vi "load_array_of_boxes_xml.vi"(8 "error in":errorcluster, 11 "node in":refnum<k20>) -> (0 "error out":errorcluster, 2 "ArrayOfDDSBoxes":T1[](array[typedef]) {"Array of DDS Channels (4)"."Array of DDS Profiles (8)"."Time Step (us)" min=0.0 max=262.14 step=0.004 format="%8.3g"; "Array of DDS Channels (4)"."Channel Parameters"."Ref Clock Rate [MHz]" min=0.0}, 3 "node":refnum<k20>)   [LabVIEW 2014, in "DDS.lvclass"]
doc: "Loads array of DDS boxes from XML. Expected format:\n\n<box>\n<Enable>%b</Enable>\n<DDSBoxDeviceReference.Resource>%s</DDSBoxDeviceReference.Resource>\n<DDSBoxDeviceReference.DIOPort>%u</DDSBoxDeviceReference.DIOPort>\n<DDSBoxDeviceReference.SerialClockRate units=\"kHz\">%u</DDSBoxDeviceReference.SerialClockRate>\n<ArrayOfDDSChannels>\n\n<channel>\n<Power>%b</Power>\n<ChannelParameters.RefClockRate units=\"kHz\">%f</ChannelParameters.RefClockRate>\n<ChannelParameters.FullScaleOutputPower units=\"dBm\">%f</ChannelParameters.FullScaleOutputPower>\n<RAMEnable>%b</RAMEnable>\n<RAMDestType>%u</RAMDestType>\n<RAMDefault.Frequency units=\"MHz\">%s</RAMDefault.Frequency>\n<RAMDefault.Amplitude units=\"dBm\">%s</RAMDefault.Amplitude>\n<RAMDefault.Phase units=\"rad\">%s</RAMDefault.Phase>\n<ArrayOfDDSProfiles>\n\n<profile>\n<SingleTone.Frequency units=\"MHz\">%s</SingleTone.Frequency>\n<SingleTone.Amplitude units=\"dBm\">%s</SingleTone.Amplitude>\n<SingleTone.Phase units=\"rad\">%s</SingleTone.Phase>\n<RAMMode>%u</RAMMode>\n<ZeroCrossing>%b</ZeroCrossing>\n<NoDwellHigh>%b</NoDwellHigh>\n<FunctionOrStatic>%b</FunctionOrStatic>\n<RAMFunctionSettings>%s</RAMFunctionSettings>\n<RAMStaticArray>%s</RAMStaticArray>\n</profile>\n\n</ArrayOfDDSProfiles>\n</channel>\n\n</ArrayOfDDSChannels>\n</box>\n\nMTL 2012 Dec 31"
uses:
  DDS.lvclass
  DDS Library/Controls/DDS RAM Mode.ctl
  DDS Library/DDS.lvlib
  <vilib>/ni845x/ni845x.llb/ni845xControl.ctl
  DDS Library/Controls/DDS Box Device Reference.ctl
  DDS Library/Controls/DDS Box Cluster.ctl
  <resource>/objmgr/DOMUserDefRef.rc
  <vilib>/xml/NI_XML.lvlib
  <vilib>/xml/Close Reference(Node).vi
  DDS Library/Controls/DDS Profile.ctl
  DDS Library/Controls/DDS Channel.ctl
  DDS Library/Controls/DDS Profile Array.ctl
  DDS Library/Controls/DDS Channel Array.ctl
  DDS Library/Controls/DDS RAM Timestep.ctl
  DDS Library/Controls/DDS RAM Destination.ctl
  DDS Library/Controls/DDS Channel Parameters.ctl
panel:
  # "f/f/A"
  # "Mag"
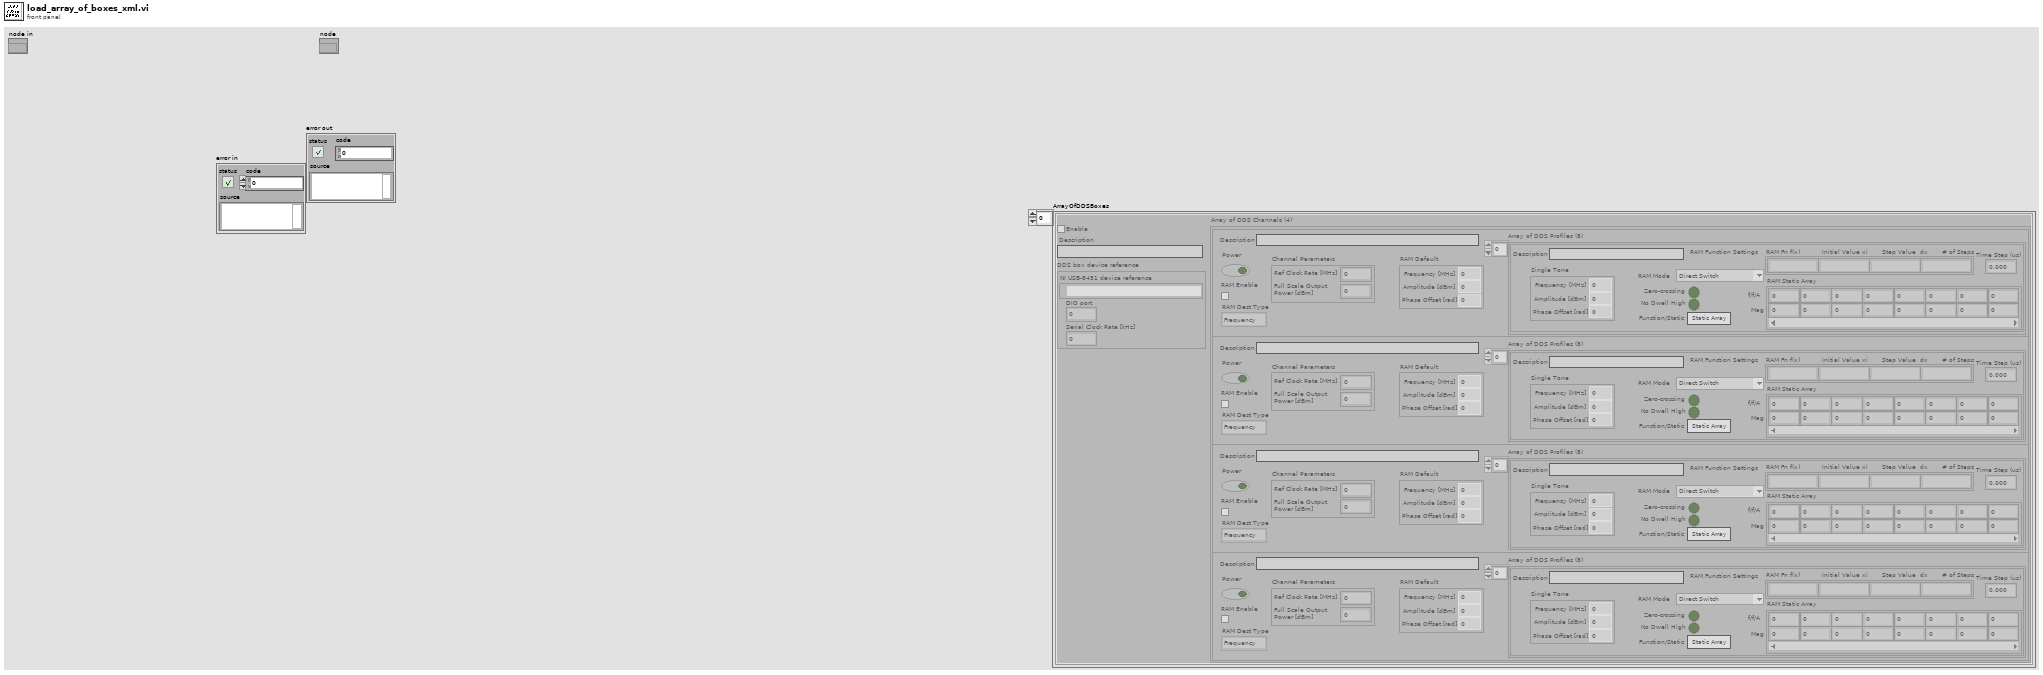
[diagram p1: front panel]
types:
  T1 = typedef "DDS.lvlib/DDS Box Cluster.ctl" = cluster{"DDS box device reference":T2, "Array of DDS Channels (4)":T4, "Enable":bool, "Description":string}
  T2 = typedef "DDS.lvlib/DDS Box Device Reference.ctl" = cluster{"NI USB-8451 device reference":T3, "DIO port":u8, "Serial Clock Rate [kHz]":u16}
  T3 = typedef "ni845xControl.ctl" = refnum<k21>
  T4 = typedef "DDS.lvlib/DDS Channel Array.ctl" = T5[]
  T5 = typedef "DDS.lvlib/DDS Channel.ctl" = cluster{"Power":bool, "Channel Parameters":T6, "RAM Enable":bool, "RAM Dest Type":T7, "RAM Default":cluster{"Frequency [MHz]":dbl, "Amplitude [dBm]":dbl, "Phase Offset [rad]":dbl}, "Array of DDS Profiles (8)":T8, "Description":string}
  T6 = typedef "DDS.lvlib/DDS Channel Parameters.ctl" = cluster{"Ref Clock Rate [MHz]":dbl, "Full Scale Output\nPower [dBm]":dbl}
  T7 = typedef "DDS.lvlib/DDS RAM Destination.ctl" = enum16{"Frequency", "Phase", "Amplitude", "Polar"}
  T8 = typedef "DDS.lvlib/DDS Profile Array.ctl" = T9[]
  T9 = typedef "DDS.lvlib/DDS Profile.ctl" = cluster{"Single Tone":cluster{"Frequency [MHz]":dbl, "Amplitude [dBm]":dbl, "Phase Offset [rad]":dbl}, "RAM Mode ":T10, "Zero-crossing":bool, "No Dwell High":bool, "Function/Static":bool, "RAM Function Settings":string[], "RAM Static Array":dbl[][], "Description":string, "Time Step (us)":T11}
  T10 = typedef "DDS.lvlib/DDS RAM mode.ctl" = enum16{"Direct Switch", "Ramp Up", "Bidirectional Ramp", "Continuous Bidirectional Ramp", "Continuous Recirculate", "Direct Switch 2", "Direct Switch 3", "Direct Switch 4"}
  T11 = typedef "DDS.lvlib/DDS RAM Timestep.ctl" = dbl
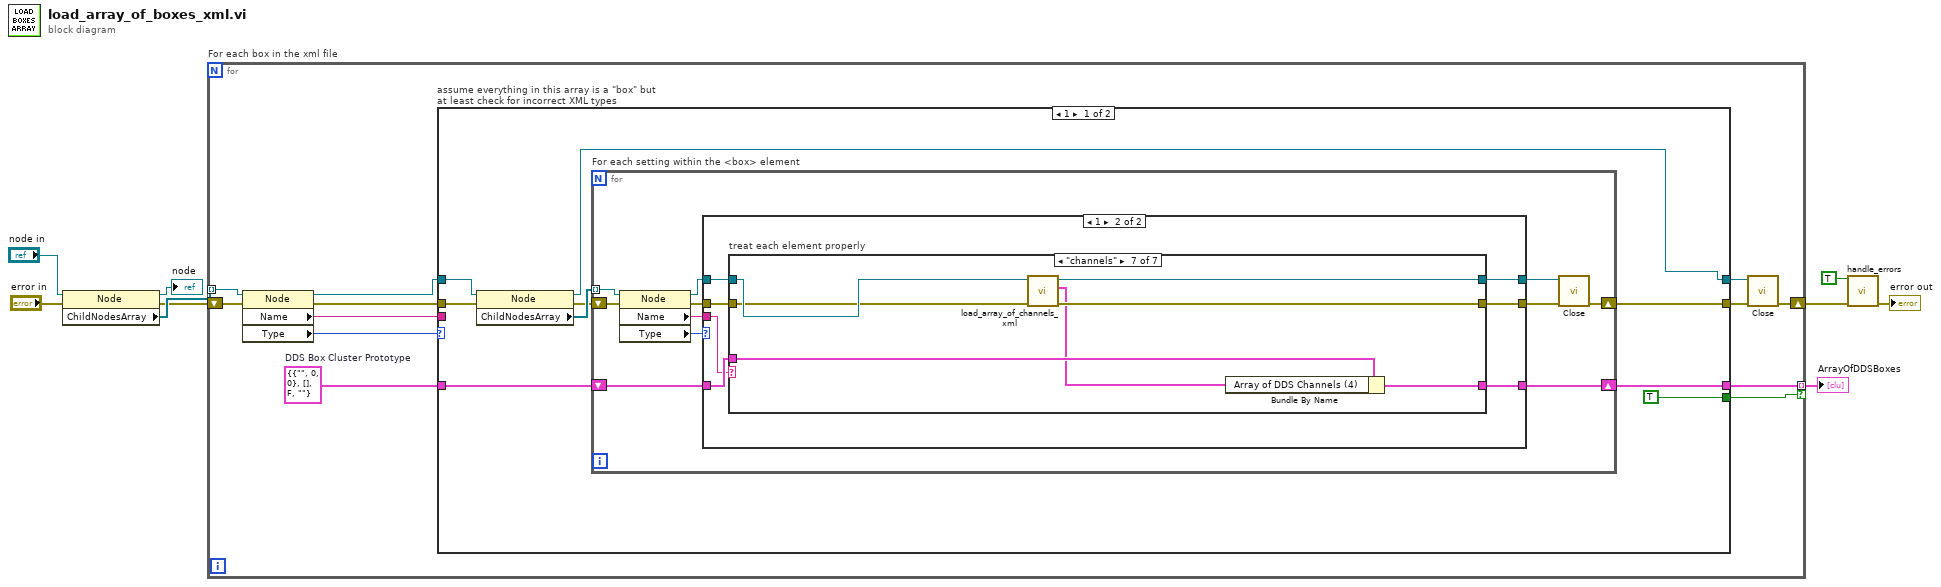
[diagram p0: block diagram]
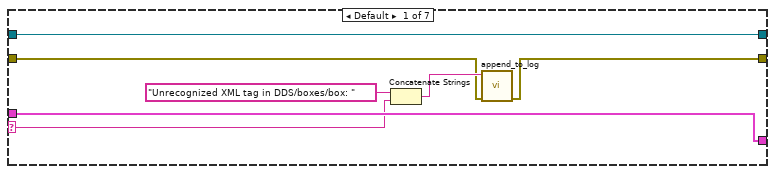
[diagram p3: hidden frame]
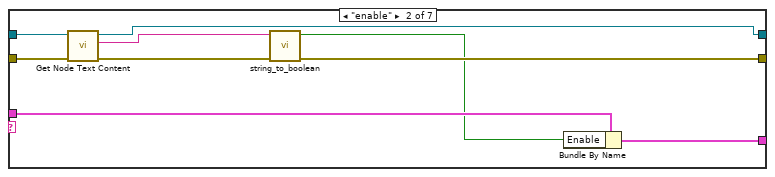
[diagram p4: hidden frame]
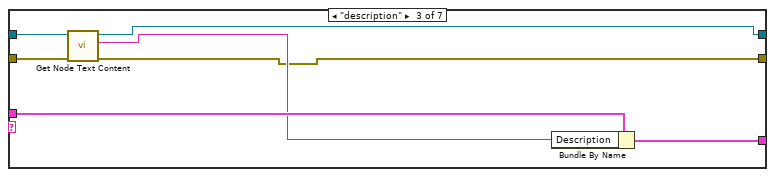
[diagram p5: hidden frame]
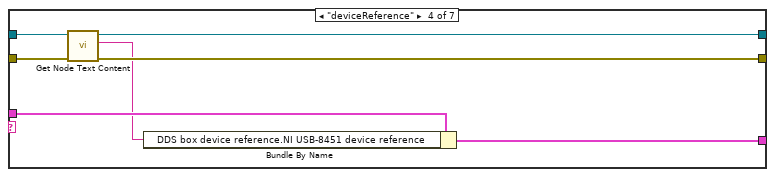
[diagram p6: hidden frame]
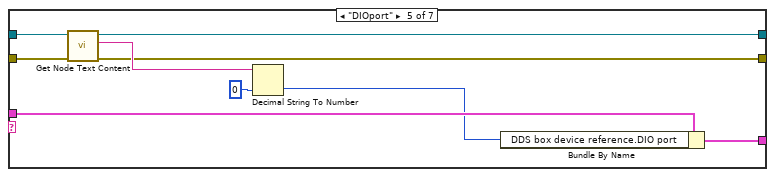
[diagram p7: hidden frame]
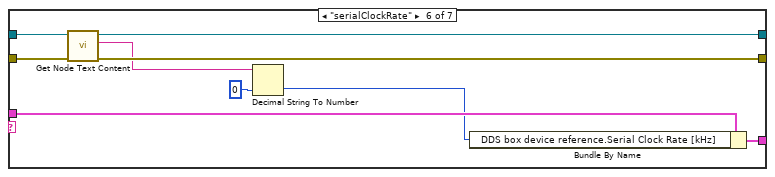
[diagram p8: hidden frame]
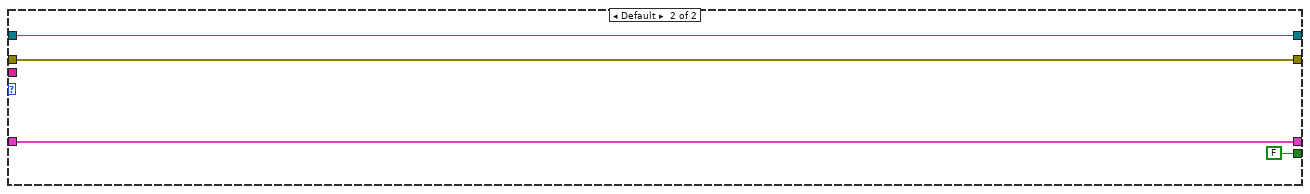
[diagram p9: hidden frame]
diagram:
  n1 = property class="Node"(reference="node in", error in="error in") -> (reference out=→"node":refnum<k20>, error out=w5:errorcluster, "ChildNodesArray"=w8:refnum<k20>[])
  n2 = for "For each box in the xml file" {
    tunnel: w8 -> [w17] mode=indexing
    shift-right: [w18] -> w4
    shift-left: w5 -> [w14]
    tunnel: [w21] -> w1 mode=indexing if=w15
    w10 = T1 {"DDS box device reference"={"NI USB-8451 device reference"="", "DIO port"=0, "Serial Clock Rate [kHz]"=0}, "Array of DDS Channels (4)"=[], "Enable"=FALSE, "Description"=""}  # DDS Box Cluster Prototype
    n3 = property class="Node"(reference=w17, error in=w14) -> (reference out=w16:refnum<k20>, error out=w13:errorcluster, "Name"=w11:string, "Type"=w12:i32)
    n4 = case "assume everything in this array is a \"box\" but at least check for incorrect XML types" shown="1" w12 {
      tunnel: [w30 w107] -> w21
      tunnel: w13 -> [w29 w110]
      tunnel: [w28 w109] -> w20
      tunnel: [w27 w110] -> w19
      tunnel: w16 -> [w26 w109]
      tunnel: [TRUE FALSE] -> w15
      tunnel: w11 -> [_ _]
      tunnel: w10 -> [w24 w107]
      frame 1 {
        n5 = property class="Node"(reference=w26, error in=w29) -> (reference out=w28:refnum<k20>, error out=w22:errorcluster, "ChildNodesArray"=w23:refnum<k20>[])
        n6 = for "For each setting within the <box> element" {
          shift-right: [w39] -> w30
          shift-left: w24 -> [w38]
          tunnel: w23 -> [w37] mode=indexing
          shift-right: [w41] -> w27
          shift-left: w22 -> [w36]
          n7 = property class="Node"(reference=w37, error in=w36) -> (reference out=w33:refnum<k20>, error out=w34:errorcluster, "Name"=w35:string, "Type"=w31:i32)
          n8 = case shown="1" w31 {
            tunnel: [w43 w51] -> w40
            tunnel: [w44 w50] -> w39
            tunnel: w38 -> [w44 w49]
            tunnel: w35 -> [_ w48]
            tunnel: w34 -> [w43 w47]
            tunnel: w33 -> [w42 w46]
            tunnel: [w42 w45] -> w32
            frame Default {
            }
            frame 1 {
              n9 = case "treat each element properly" shown="\"channels\"" w48 {
                selector: w48 -> [w52 _ _ _ _ _ _]
                tunnel: w47 -> [w54 w64 w71 w78 w83 w94 w102]
                tunnel: [w53 w60 w68 w77 w82 w93 w104] -> w51
                tunnel: w49 -> [w58 w67 w74 w81 w90 w99 w106]
                tunnel: [w58 w66 w73 w80 w89 w98 w105] -> w50
                tunnel: w46 -> [w57 w65 w72 w79 w86 w95 w103]
                tunnel: [w57 w63 w70 w76 w85 w92 w100] -> w45
                frame Default {
                  n10 = Concatenate Strings("Unrecognized XML tag in DDS/boxes/box: " ("string"), w52) -> (w55:string)
                  n11 = call "append_to_log.vi"("error in"=w54, "string"=w55) -> ("error out"=w53:errorcluster)  [unwired: 9 in]
                }
                frame "enable" {
                  n12 = call <vilib>:"Get Node Text Content.vi"("error in (no error)"=w64, "node in"=w65) -> ("error out"=w61:errorcluster, "node text"=w62:string, "node out"=w63:refnum<k20>)  [unwired: 7 in]
                  n13 = call "string_to_boolean.vi"("error in"=w61, "string"=w62) -> ("error out"=w60:errorcluster, "boolean"=w59:bool)  [unwired: 8 in]
                  n14 = Bundle By Name(cluster=w67, "Enable"=w59) -> (w66:T1)
                }
                frame "description" {
                  n15 = call <vilib>:"Get Node Text Content.vi"("error in (no error)"=w71, "node in"=w72) -> ("error out"=w68:errorcluster, "node text"=w69:string, "node out"=w70:refnum<k20>)  [unwired: 7 in]
                  n16 = Bundle By Name(cluster=w74, "Description"=w69) -> (w73:T1)
                }
                frame "deviceReference" {
                  n17 = call <vilib>:"Get Node Text Content.vi"("error in (no error)"=w78, "node in"=w79) -> ("error out"=w77:errorcluster, "node text"=w75:string, "node out"=w76:refnum<k20>)  [unwired: 7 in]
                  n18 = Bundle By Name(cluster=w81, "DDS box device reference.NI USB-8451 device reference"=w75) -> (w80:T1)
                }
                frame "DIOport" {
                  n19 = call <vilib>:"Get Node Text Content.vi"("error in (no error)"=w83, "node in"=w86) -> ("error out"=w82:errorcluster, "node text"=w84:string, "node out"=w85:refnum<k20>)  [unwired: 7 in]
                  n20 = Decimal String To Number(string=w84, default (0L)=u8 0 ("default (0 I32)")) -> (number=w87:u8)  [unwired: 1 in, 1 out]
                  n21 = Bundle By Name(cluster=w90, "DDS box device reference.DIO port"=w87) -> (w89:T1)
                }
                frame "serialClockRate" {
                  n22 = call <vilib>:"Get Node Text Content.vi"("error in (no error)"=w94, "node in"=w95) -> ("error out"=w93:errorcluster, "node text"=w91:string, "node out"=w92:refnum<k20>)  [unwired: 7 in]
                  n23 = Decimal String To Number(string=w91, default (0L)=u16 0 ("default (0 I32)")) -> (number=w97:u16)  [unwired: 1 in, 1 out]
                  n24 = Bundle By Name(cluster=w99, "DDS box device reference.Serial Clock Rate [kHz]"=w97) -> (w98:T1)
                }
                frame "channels" {
                  n25 = call "load_array_of_channels_xml.vi"("error in"=w102, "node in"=w103) -> ("error out"=w104:errorcluster, "Array of DDS Channels (4)"=w101:T4, "node"=w100:refnum<k20>)  [unwired: 7 in]
                  n26 = Bundle By Name(cluster=w106, "Array of DDS Channels (4)"=w101) -> (w105:T1)
                }
              }
            }
          }
          n27 = call-poly <vilib>:"Close.vi"("error in (no error)"=w40, "node"=w32) -> ("error out"=w41:errorcluster)  [unwired: 7 in]
        }
      }
      frame Default {
      }
    }
    n28 = call-poly <vilib>:"Close.vi"("error in (no error)"=w19, "node"=w20) -> ("error out"=w18:errorcluster)  [unwired: 7 in]
  }
  "ArrayOfDDSBoxes" <- w1
  n29 = call "handle_errors.vi"("Exit Operation"=TRUE, "error in (no error)"=w4) -> ("error out"=→"error out":errorcluster)  [unwired: 13 in]
